vi "RichToFlatnixnet_grpc_ConvertByteArrayToFramesSinglePointRequest.vi"(5 "OutputClusterType":T1, 11 "InputCluster":T4) -> (3 "OutputCluster":T1)   [LabVIEW 2025, in "grpc-xnet_client.lvlib"]
uses:
  grpc-xnet_client.lvlib
  nixnet_grpc_ConvertByteArrayToFramesSinglePointRequest.ctl
  nixnet_grpc_ConvertByteArrayToFramesSinglePointRequest_protocol_enum/nixnet_grpc_ConvertByteArrayToFramesSinglePointRequest_protocol_enum.lvclass
  nidevice_grpc_Session.ctl
  nixnet_grpc_ConvertByteArrayToFramesSinglePointRequest_Flat.ctl
  nidevice_grpc_Session_Flat.ctl
  nixnet_grpc_Protocol.ctl
  nixnet_grpc_ConvertByteArrayToFramesSinglePointRequest_protocol_enum/nixnet_grpc_ConvertByteArrayToFramesSinglePointRequest_protocol_enum.lvclass/nixnet_grpc_ConvertByteArrayToFramesSinglePointRequest_protocol_enum.ctl
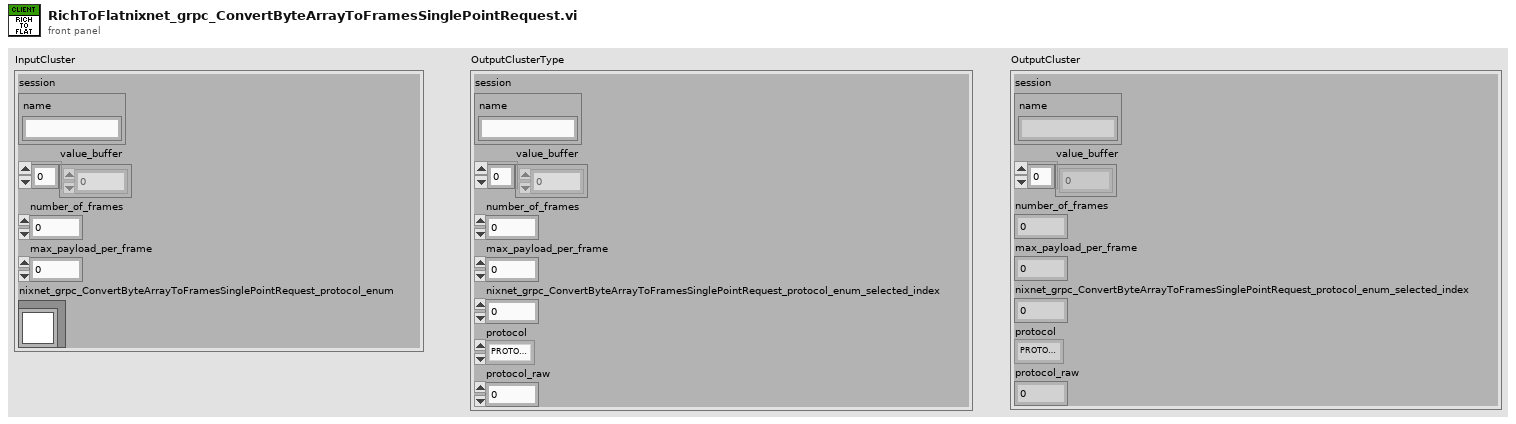
[diagram p1: front panel]
types:
  T1 = typedef "grpc-xnet_client.lvlib/nixnet_grpc_ConvertByteArrayToFramesSinglePointRequest_Flat.ctl" = cluster{"session":T2, "value_buffer":u8[], "number_of_frames":u32, "max_payload_per_frame":u32, "nixnet_grpc_ConvertByteArrayToFramesSinglePointRequest_protocol_enum_selected_index":i32, "protocol":T3, "protocol_raw":u32}
  T2 = typedef "grpc-xnet_client.lvlib/nidevice_grpc_Session_Flat.ctl" = cluster{"name":string}
  T3 = typedef "grpc-xnet_client.lvlib/nixnet_grpc_Protocol.ctl" = enum32{"PROTOCOL_UNSPECIFIED", "PROTOCOL_CAN", "PROTOCOL_LIN", "PROTOCOL_FLEX_RAY", "PROTOCOL_J1939", "PROTOCOL_ENET"}
  T4 = typedef "grpc-xnet_client.lvlib/nixnet_grpc_ConvertByteArrayToFramesSinglePointRequest.ctl" = cluster{"session":T5, "value_buffer":u8[], "number_of_frames":u32, "max_payload_per_frame":u32, "nixnet_grpc_ConvertByteArrayToFramesSinglePointRequest_protocol_enum":refnum<class "nixnet_grpc_ConvertByteArrayToFramesSinglePointRequest_protocol_enum.lvclass">}
  T5 = typedef "grpc-xnet_client.lvlib/nidevice_grpc_Session.ctl" = cluster{"name":string}
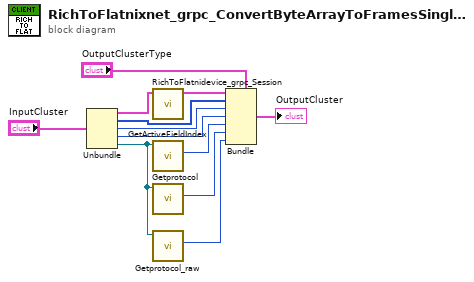
[diagram p0: block diagram]
diagram:
  n1 = Unbundle "Unbundle"("InputCluster") -> ("session"=w9:T5, "value_buffer"=w7:u8[], "number_of_frames"=w6:u32, "max_payload_per_frame"=w5:u32, "nixnet_grpc_ConvertByteArrayToFramesSinglePointRequest_protocol_enum"=w4:refnum<class "nixnet_grpc_ConvertByteArrayToFramesSinglePointRequest_protocol_enum.lvclass">)
  n2 = call "RichToFlatnidevice_grpc_Session.vi"("InputCluster"=w9) -> ("OutputCluster"=w8:T2)  [unwired: 10 in]
  n3 = call "GetActiveFieldIndex.vi"("OneOfTemplate in"=w4) -> ("Active Field Index"=w3:i32)  [unwired: 8 in, 2 out]
  n4 = call "Getprotocol.vi"("OneOfTemplate in"=w4) -> ("Get_Val"=w2:T3)  [unwired: 8 in, 2 out]
  n5 = call "Getprotocol_raw.vi"("OneOfTemplate in"=w4) -> ("Get_Val"=w1:u32)  [unwired: 8 in, 2 out]
  n6 = Bundle "Bundle"(cluster="OutputClusterType", "session"=w8, "value_buffer"=w7, "number_of_frames"=w6, "max_payload_per_frame"=w5, "nixnet_grpc_ConvertByteArrayToFramesSinglePointRequest_protocol_enum_selected_index"=w3, "protocol"=w2, "protocol_raw"=w1) -> (→"OutputCluster":T1)
